vi "Async Loop Control.vi"(0 "RT Data In":T1 {"End System Handle" format="%x"; "Label Transfer Config"."Block Data Refs"."Data Reference" format="%.0x"; "Status Config"."Hardware Out Dur Reference" format="%.0x"; "Status Config"."Hardware In Dur Reference" format="%.0x"; "Status Config"."Hardware Out Count Reference" format="%.0x"; "Status Config"."Hardware In Count Reference" format="%.0x"; "Status Config"."Error Data Reference" format="%.0x"; "Hardware Output Tx Channels"."Message Settings"."Transmit Channel Data Reference" format="%.0x"; "Hardware Output Tx Channels"."Message Settings"."Queue Transmit Channel" format="%.0x"; "Hardware Output Tx Channels"."Message Settings"."Driver Data"."Num Bits" min=1 max=32; "Hardware Output Tx Channels"."Message Settings"."Block Data Refs"."Data Reference" format="%.0x"; "Hardware Output Tx Channels"."Rx Com Udp Port"."Handle" format="%08x"; "Hardware Output Tx Channels"."Tx Com Udp Port"."Handle" format="%08x"; "Hardware Input Rx Channels"."Message Settings"."Transmit Channel Data Reference" format="%.0x"; "Hardware Input Rx Channels"."Message Settings"."Queue Transmit Channel" format="%.0x"; "Hardware Input Rx Channels"."Message Settings"."Driver Data"."Num Bits" min=1 max=32; "Hardware Input Rx Channels"."Message Settings"."Block Data Refs"."Data Reference" format="%.0x"; "Hardware Input Rx Channels"."Rx Com Udp Port"."Handle" format="%08x"; "Hardware Input Rx Channels"."Tx Com Udp Port"."Handle" format="%08x"}, 2 "Action":T17, 11 "error in (no error)":errorcluster) -> (4 "RT Data Out":T1 {"End System Handle" format="%x"; "Label Transfer Config"."Block Data Refs"."Data Reference" format="%.0x"; "Status Config"."Hardware Out Dur Reference" format="%.0x"; "Status Config"."Hardware In Dur Reference" format="%.0x"; "Status Config"."Hardware Out Count Reference" format="%.0x"; "Status Config"."Hardware In Count Reference" format="%.0x"; "Status Config"."Error Data Reference" format="%.0x"; "Hardware Output Tx Channels"."Message Settings"."Transmit Channel Data Reference" format="%.0x"; "Hardware Output Tx Channels"."Message Settings"."Queue Transmit Channel" format="%.0x"; "Hardware Output Tx Channels"."Message Settings"."Driver Data"."Num Bits" min=1 max=32; "Hardware Output Tx Channels"."Message Settings"."Block Data Refs"."Data Reference" format="%.0x"; "Hardware Output Tx Channels"."Rx Com Udp Port"."Handle" format="%08x"; "Hardware Output Tx Channels"."Tx Com Udp Port"."Handle" format="%08x"; "Hardware Input Rx Channels"."Message Settings"."Transmit Channel Data Reference" format="%.0x"; "Hardware Input Rx Channels"."Message Settings"."Queue Transmit Channel" format="%.0x"; "Hardware Input Rx Channels"."Message Settings"."Driver Data"."Num Bits" min=1 max=32; "Hardware Input Rx Channels"."Message Settings"."Block Data Refs"."Data Reference" format="%.0x"; "Hardware Input Rx Channels"."Rx Com Udp Port"."Handle" format="%08x"; "Hardware Input Rx Channels"."Tx Com Udp Port"."Handle" format="%08x"}, 15 "error out":errorcluster)   [LabVIEW 2014, in "AIT 664 Custom Device.lvlib"]
doc: "Controls the Async Loops according to the action input."
uses:
  AIT 664 Custom Device.lvlib
  RT Controls/AIT 664  - RT Data.ctl
  RT Controls/AIT 664 - RT Hardware Channel.ctl
  RT Controls/AIT 664 - RT Message Settings.ctl
  <vilib>/NI Veristand/Custom Device API/Block Data Reference.ctl
  <vilib>/NI Veristand/Custom Device API/Data Reference.ctl
  RT Controls/AIT 664 - Driver Data.ctl
  Controls and Global/Start Bit.ctl
  Controls and Global/Number of Bits.ctl
  <vilib>/NI Veristand/Custom Device API/Custom Device Item Ref.ctl
  <userlib>/ARINC 664/AIT 664 Controls/General/Message Port.ctl
  <userlib>/ARINC 664/AIT 664 Controls/General/Direction.ctl
  <userlib>/ARINC 664/AIT 664 Controls/General/Message Port Type.ctl
  System Explorer/Controls/664 - Sampling Type.ctl
  RT Controls/Status Channels Config.ctl
  RT Controls/FIFO.ctl
  RT Controls/Label Transfer Config.ctl
  RT Controls/Async Loop Control Enum.ctl
  <vilib>/NI Veristand/Custom Device Tools/Custom Device Utility Library/Custom Device Utility Library.lvlib
  <vilib>/NI Veristand/Custom Device API/Custom Device API.lvlib
  <userlib>/ARINC 664/AIT 664 API.lvlib
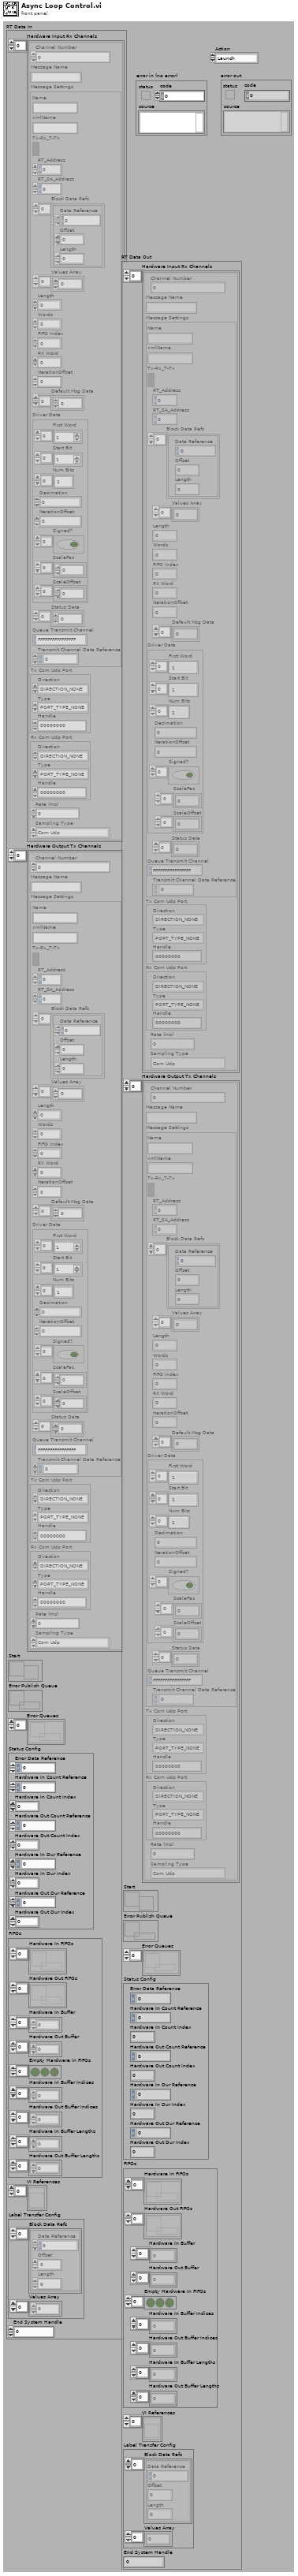
[diagram p1: front panel]
types:
  T1 = typedef "AIT 664 Custom Device.lvlib/AIT 664  - RT Data.ctl" = cluster{"Hardware Input Rx Channels":T2[], "Hardware Output Tx Channels":T2[], "Start":refnum<notifier>, "Error Publish Queue":refnum<queue>, "Error Queues":refnum<queue>[], "Status Config":T14, "FIFOs":T15, "VI References":refnum<vi>[], "Label Transfer Config":T16, "End System Handle ":u64}
  T2 = typedef "AIT 664 Custom Device.lvlib/AIT 664 - RT Hardware Channel.ctl" = cluster{"Channel Number":u16, "Message Name":string, "Message Settings":T3, "Tx Com Udp Port":T10, "Rx Com Udp Port":T10, "Rate (ms)":u32, "Sampling Type":T13}
  T3 = typedef "AIT 664 Custom Device.lvlib/AIT 664 - RT Message Settings.ctl" = cluster{"Name":string, "xmlName":string, "Tx-Rx_T-Tx":bool, "RT_Address":u8, "RT_SA_Address":u8, "Block Data Refs":T4[], "Values Array":dbl[], "Length":i32, "Words":i32, "FIFO Index":i32, "RX Word":u32, "IterationOffset":i32, "Default Msg Data":u8[], "Driver Data":T6, "Status Data":u32[], "Queue Transmit Channel":T9, "Transmit Channel Data Reference":T5}
  T4 = typedef "Custom Device API.lvlib/Block Data Reference.ctl" = cluster{"Data Reference":T5, "Offset":i32, "Length":i32}
  T5 = typedef "Custom Device API.lvlib/Data Reference.ctl" = i32
  T6 = typedef "AIT 664 Custom Device.lvlib/AIT 664 - Driver Data.ctl" = cluster{"First Word":T7[], "Start Bit":T7[], "Num Bits":T8[], "Decimation":i32, "IterationOffset":i32, "Signed?":bool[], "ScaleFac":dbl[], "ScaleOffset":dbl[]}
  T7 = typedef "AIT 664 Custom Device.lvlib/Start Bit.ctl" = i32
  T8 = typedef "AIT 664 Custom Device.lvlib/Number of Bits.ctl" = i32
  T9 = typedef "Custom Device API.lvlib/Custom Device Item Ref.ctl" = u64
  T10 = typedef "AIT 664 API.lvlib/Message Port.ctl" = cluster{"Direction":T11, "Type":T12, "Handle":u64}
  T11 = typedef "AIT 664 API.lvlib/Direction.ctl" = enum16{"DIRECTION_NONE", "DIRECTION_TX", "DIRECTION_RX"}
  T12 = typedef "AIT 664 API.lvlib/Message Port Type.ctl" = enum16{"PORT_TYPE_NONE", "COM_UDP", "SAP_UDP", "SAP_IP", "SAP_MAC", "COTS_MAC", "COTS_MAC_RAW"}
  T13 = typedef "AIT 664 Custom Device.lvlib/664 - Sampling Type.ctl" = enum16{"Com Udp", "Com Udp Queuing", "Sap Udp", "Sap Ip", "Sap Mac", "Unknown"}
  T14 = typedef "AIT 664 Custom Device.lvlib/Status Channels Config.ctl" = cluster{"Error Data Reference":T5, "Hardware In Count Reference":T5, "Hardware In Count Index":i32, "Hardware Out Count Reference":T5, "Hardware Out Count Index":i32, "Hardware In Dur Reference":T5, "Hardware In Dur Index":i32, "Hardware Out Dur Reference":T5, "Hardware Out Dur Index":i32}
  T15 = typedef "AIT 664 Custom Device.lvlib/FIFO.ctl" = cluster{"Hardware In FIFOs":refnum<k33>[], "Hardware Out FIFOs":refnum<k33>[], "Hardware In Buffer":dbl[], "Hardware Out Buffer":dbl[], "Empty Hardware In FIFOs":bool[], "Hardware In Buffer Indices":i32[], "Hardware Out Buffer Indices":i32[], "Hardware In Buffer Lengths":i32[], "Hardware Out Buffer Lengths":i32[]}
  T16 = typedef "AIT 664 Custom Device.lvlib/Label Transfer Config.ctl" = cluster{"Block Data Refs":T4[], "Values Array":dbl[]}
  T17 = typedef "AIT 664 Custom Device.lvlib/Async Loop Control Enum.ctl" = enum16{"Launch", "Start", "Stop"}
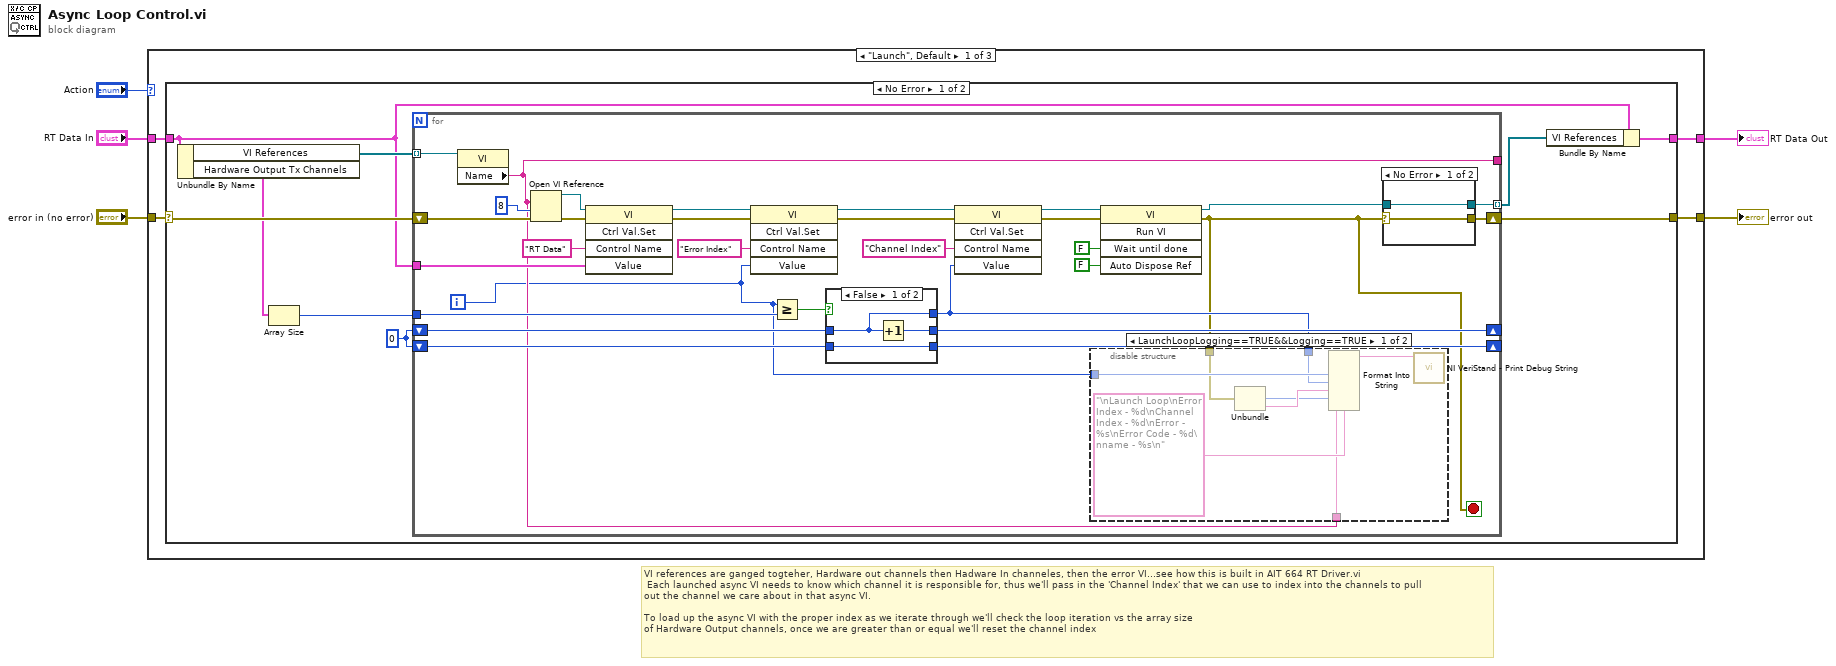
[diagram p0: block diagram]
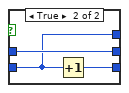
[diagram p3: hidden frame]
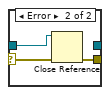
[diagram p4: hidden frame]
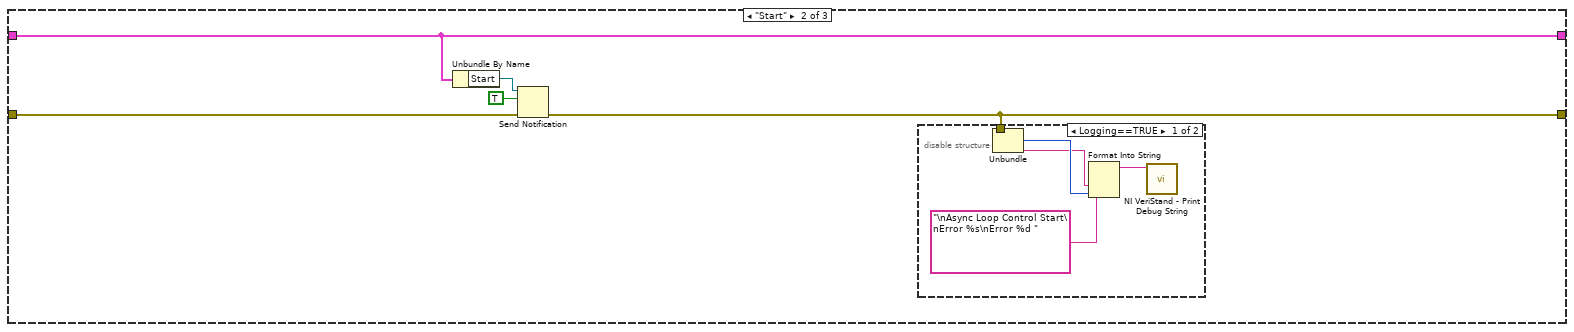
[diagram p6: hidden frame]
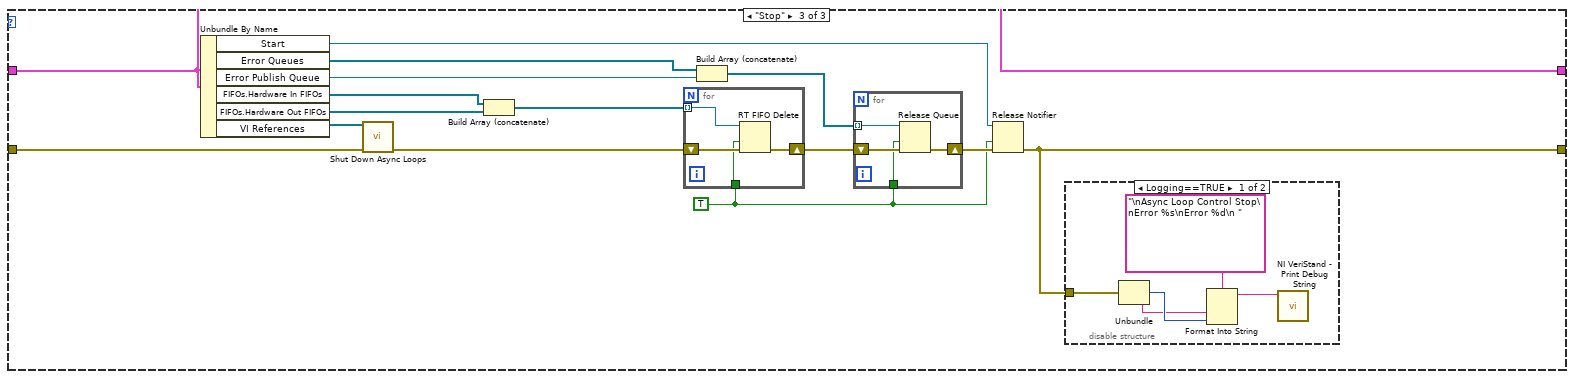
[diagram p8: hidden frame]
diagram:
  # "VI references are ganged togteher, Hardware out channels then Hadware In channeles, then the error VI...see how this is built in AIT 664 RT Driver.vi\n Each launched async VI needs to know which channel it is responsible for, thus we'll pass in the 'Channel Index' that we can use to index into the channels to pull\nout the channel we care about in that async VI.\n\nTo load up the async VI with the proper index as we iterate through we'll check the loop iteration vs the array size\nof Hardware Output channels, once we are greater than or equal we'll reset the channel index"
  n1 = case shown="\"Launch\", Default" "Action" {
    tunnel: [w9 w70 w81] -> w5
    tunnel: "error in (no error)" -> [w8 w73 w84]
    tunnel: "RT Data In" -> [w7 w71 w87]
    tunnel: [w6 w71 w87] -> w1
    frame "Launch", Default {
      n2 = case shown="No Error" w8 {
        selector: w8 -> [w18 w69]
        tunnel: [w10 w69] -> w9
        tunnel: w7 -> [w14 w68]
        tunnel: [w15 w68] -> w6
        frame No Error {
          w11 = 0
          n3 = Unbundle By Name(w14) -> ("VI References"=w17:refnum<vi>[], "Hardware Output Tx Channels"=w13:T2[])
          n4 = Array Size(array=w13) -> (size(s)=w12:i32)
          n5 = for {
            shift-right: [w23] -> w10
            shift-left: w18 -> [w48]
            tunnel: w17 -> [w47] mode=indexing
            tunnel: w14 -> [w39]
            tunnel: [w46] -> w16 mode=indexing
            shift-right: [w29] -> _
            shift-left: w11 -> [w30]
            tunnel: w12 -> [w24]
            shift-right: [w27] -> _
            shift-left: w11 -> [w28]
            tunnel: [w21] -> _
            i -> [w20]
            stop <- w22 stop-if-true
            n6 = property class="VI"(reference=w47) -> ("Name"=w21:string)  [unwired: 1 in, 2 out]
            n7 = Open VI Reference(vi path=w21, options=8, error in (no error)=w48) -> (vi reference=w25:refnum<vi>, error out=w41:errorcluster)  [unwired: 3 out]
            n8 = invoke class="VI" method="Ctrl Val.Set"(reference=w25, error in=w41, "Control Name"="RT Data", "Value"=w39) -> (reference out=w19:refnum<vi>, error out=w38:errorcluster)  [unwired: 1 in, 3 out]
            n9 = invoke class="VI" method="Ctrl Val.Set"(reference=w19, error in=w38, "Control Name"="Error Index", "Value"=w20) -> (reference out=w37:refnum<vi>, error out=w35:errorcluster)  [unwired: 1 in, 3 out]
            n10 = Greater Or Equal?(x=w20, y=w24) -> (x >= y?=w31:bool)
            n11 = case shown="False" w31 {
              tunnel: w30 -> [w59 w62]
              tunnel: [w59 w61] -> w26
              tunnel: [w58 w62] -> w29
              tunnel: w28 -> [w57 w61]
              tunnel: [w57 w60] -> w27
              frame False {
                n12 = Increment(x=w59) -> (x+1=w58:i32)
              }
              frame True {
                n13 = Increment(x=w61) -> (x+1=w60:i32)
              }
            }
            n14 = invoke class="VI" method="Ctrl Val.Set"(reference=w37, error in=w35, "Control Name"="Channel Index", "Value"=w26) -> (reference out=w36:refnum<vi>, error out=w34:errorcluster)  [unwired: 1 in, 3 out]
            n15 = invoke class="VI" method="Run VI"(reference=w36, error in=w34, "Wait until done"=FALSE ("Wait Until Done"), "Auto Dispose Ref"=FALSE ("Auto Dispose Reference")) -> (reference out=w42:refnum<vi>, error out=w22:errorcluster)  [unwired: 1 in, 3 out]
            n16 = disable-structure shown="LaunchLoopLogging==TRUE&&Logging==TRUE" {
              disable-tunnel: w20 -> [w55 _]
              disable-tunnel: w26 -> [w54 _]
              disable-tunnel: w22 -> [w53 _]
              disable-tunnel: w21 -> [w50 _]
              frame condition #0 {
                n17 = Unbundle(w53) -> ("code"=w51:i32, "source"=w52:string)  [unwired: 1 out]
                n18 = Format Into String(format string="\nLaunch Loop\nError Index - %d\nChannel Index - %d\nError - %s\nError Code - %d\nname - %s\n", w55, w54, w52, w51, w50) -> (resulting string=w49:string)  [unwired: 2 in, 1 out]
                n19 = call <vilib>:"NI VeriStand - Print Debug String.vi"("Message"=w49) -> ()  [unwired: 10 in, 1 out]
              }
              frame condition #1 (active) {
              }
            }
            n20 = case shown="No Error" w22 {
              selector: w22 -> [w64 w67]
              tunnel: w42 -> [w63 w66]
              tunnel: [w64 w65] -> w23
              tunnel: [w63 _] -> w46
              frame No Error {
              }
              frame Error {
                n21 = Close Reference(reference=w66, error in (no error)=w67) -> (error out=w65:errorcluster)
              }
            }
          }
          n22 = Bundle By Name(cluster=w14, "VI References"=w16) -> (w15:T1)
        }
        frame Error {
        }
      }
    }
    frame "Start" {
      n23 = Unbundle By Name(w71) -> ("Start"=w74:refnum<notifier>)
      n24 = Send Notification(notification=TRUE, notifier=w74, error in (no error)=w73) -> (error out=w70:errorcluster)  [unwired: 1 out]
      n25 = disable-structure shown="Logging==TRUE" {
        disable-tunnel: w70 -> [w78 _]
        frame condition #0 (active) {
          n26 = Unbundle(w78) -> ("code"=w77:i32, "source"=w76:string)  [unwired: 1 out]
          n27 = Format Into String(format string="\nAsync Loop Control Start\nError %s\nError %d ", w76, w77) -> (resulting string=w75:string)  [unwired: 2 in, 1 out]
          n28 = call <vilib>:"NI VeriStand - Print Debug String.vi"("Message"=w75) -> ()  [unwired: 10 in, 1 out]
        }
        frame condition #1 {
        }
      }
    }
    frame "Stop" {
      w88 = TRUE ("force destroy? (F)")
      n29 = Unbundle By Name(w87) -> ("Start"=w92:refnum<notifier>, "Error Queues"=w80:refnum<queue>[], "Error Publish Queue"=w94:refnum<queue>, "FIFOs.Hardware In FIFOs"=w91:refnum<k33>[], "FIFOs.Hardware Out FIFOs"=w85:refnum<k33>[], "VI References"=w82:refnum<vi>[])
      n30 = call "Shut Down Async Loops.vi"("VI Refs"=w82, "error in (no error)"=w84) -> ("error out"=w83:errorcluster)  [unwired: 13 in]
      n31 = Build Array (concatenate)(w91, w85) -> (w90:refnum<k33>[])
      n32 = for {
        shift-right: [w102] -> w89
        shift-left: w83 -> [w103]
        tunnel: w90 -> [w101] mode=indexing
        tunnel: w88 -> [w100]
        n33 = RT FIFO Delete(0:w101, 2:w100, 3:w103) -> (11:w102:errorcluster)
      }
      n34 = Build Array (concatenate)(w80, w94) -> (w86:refnum<queue>[])
      n35 = for {
        shift-right: [w106] -> w93
        shift-left: w89 -> [w107]
        tunnel: w86 -> [w105] mode=indexing
        tunnel: w88 -> [w104]
        n36 = Release Queue(queue=w105, force destroy? (F)=w104, error in (no error)=w107) -> (error out=w106:errorcluster)  [unwired: 2 out]
      }
      n37 = Release Notifier(notifier=w92, force destroy? (F)=w88, error in (no error)=w93) -> (error out=w81:errorcluster)  [unwired: 2 out]
      n38 = disable-structure shown="Logging==TRUE" {
        disable-tunnel: w81 -> [w96 _]
        frame condition #0 (active) {
          n39 = Unbundle(w96) -> ("code"=w98:i32, "source"=w97:string)  [unwired: 1 out]
          n40 = Format Into String(format string="\nAsync Loop Control Stop\nError %s\nError %d\n ", w97, w98) -> (resulting string=w95:string)  [unwired: 2 in, 1 out]
          n41 = call <vilib>:"NI VeriStand - Print Debug String.vi"("Message"=w95) -> ()  [unwired: 10 in, 1 out]
        }
        frame condition #1 {
        }
      }
    }
  }
  "error out" <- w5
  "RT Data Out" <- w1
